vi "Configure Trigger.vi"(7 "Trigger Slope (0: Positive)":u16(ring) items=["Positive", "Negative"], 8 "error in (no error)":errorcluster, 9 "Trigger Level (1)":dbl=1.0, 10 "Trigger Source (0: Immediate)":u16(ring) items=["Immediate", "Software", "External", "Video"], 11 "VISA resource name":refnum<visa-resource-name>) -> (0 "error out":errorcluster, 3 "VISA resource name out":refnum<visa-resource-name>)   [LabVIEW 2015, in "Template - Spectrum Analyzer.lvlib"]
doc: "Configures the trigger settings on the spectrum analyzer."
uses:
  <instrlib>/_Template - Spectrum Analyzer/Template - Spectrum Analyzer.lvlib
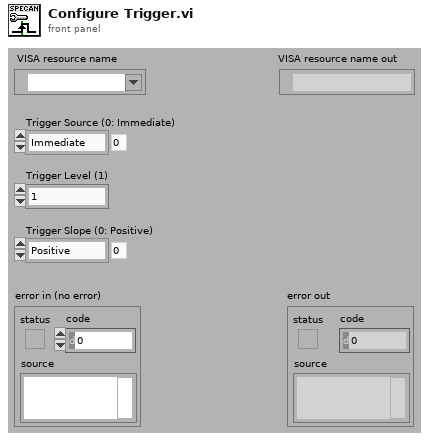
[diagram p1: front panel]
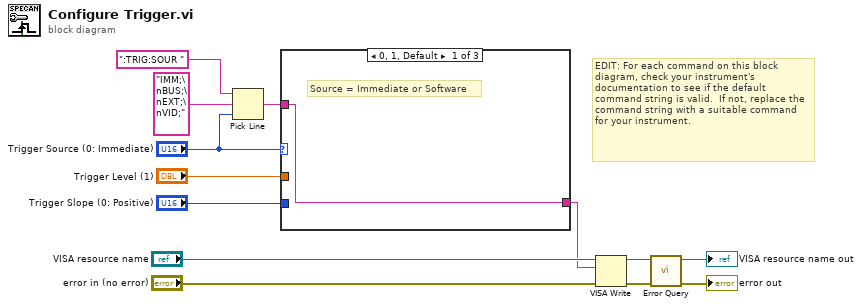
[diagram p0: block diagram]
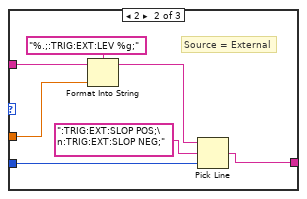
[diagram p2: hidden frame]
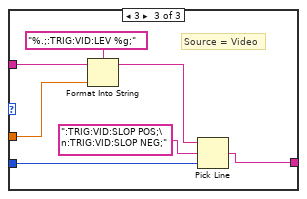
[diagram p3: hidden frame]
diagram:
  # "EDIT: For each command on this block diagram, check your instrument's documentation to see if the default command string is valid.  If not, replace the command string with a suitable command for your instrument."
  n1 = Pick Line(string ("")=":TRIG:SOUR ", multi-line string="IMM;\nBUS;\nEXT;\nVID;", line index="Trigger Source (0: Immediate)") -> (output string=w9:string)
  n2 = case shown="0, 1, Default" "Trigger Source (0: Immediate)" {
    tunnel: w9 -> [w14 w15 w28]
    tunnel: "Trigger Level (1)" -> [_ w16 w26]
    tunnel: [w14 w18 w22] -> w8
    tunnel: "Trigger Slope (0: Positive)" -> [_ w17 w23]
    frame 0, 1, Default {
      # "Source = Immediate or Software"
    }
    frame 2 {
      # "Source = External"
      n3 = Format Into String(format string="%.;:TRIG:EXT:LEV %g;", initial string=w15, w16) -> (resulting string=w19:string)  [unwired: 1 in, 1 out]
      n4 = Pick Line(string ("")=w19, multi-line string=":TRIG:EXT:SLOP POS;\n:TRIG:EXT:SLOP NEG;", line index=w17) -> (output string=w18:string)
    }
    frame 3 {
      # "Source = Video"
      n5 = Format Into String(format string="%.;:TRIG:VID:LEV %g;", initial string=w28, w26) -> (resulting string=w24:string)  [unwired: 1 in, 1 out]
      n6 = Pick Line(string ("")=w24, multi-line string=":TRIG:VID:SLOP POS;\n:TRIG:VID:SLOP NEG;", line index=w23) -> (output string=w22:string)
    }
  }
  n7 = VISA Write(VISA resource name="VISA resource name", write buffer=w8, error in (no error)="error in (no error)") -> (VISA resource name out=w4:refnum<visa-resource-name>, error out=w2:errorcluster)  [unwired: 1 out]
  n8 = call <instrlib>:"Error Query.vi"("error in (no error)"=w2, "VISA resource name"=w4) -> ("error out"=→"error out":errorcluster, "VISA resource name out"=→"VISA resource name out":refnum<visa-resource-name>)  [unwired: 6 in, 2 out]
